vi "test compare float.vi"(8 "error in (no error)":errorcluster, 11 "VI Tester Test in":refnum<class "VI Tester Test 14.lvclass">) -> (0 "error out":errorcluster, 3 "VI Tester Test out":refnum<class "VI Tester Test 14.lvclass">)   [LabVIEW 2020, in "VI Tester Test 14.lvclass"]
uses:
  VI Tester Test 14.lvclass
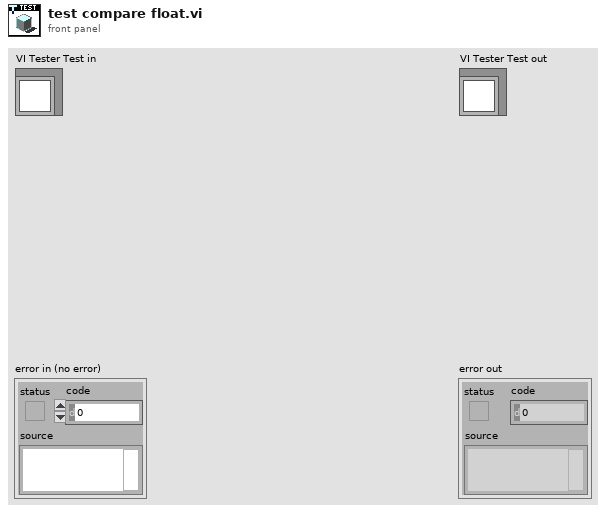
[diagram p1: front panel]
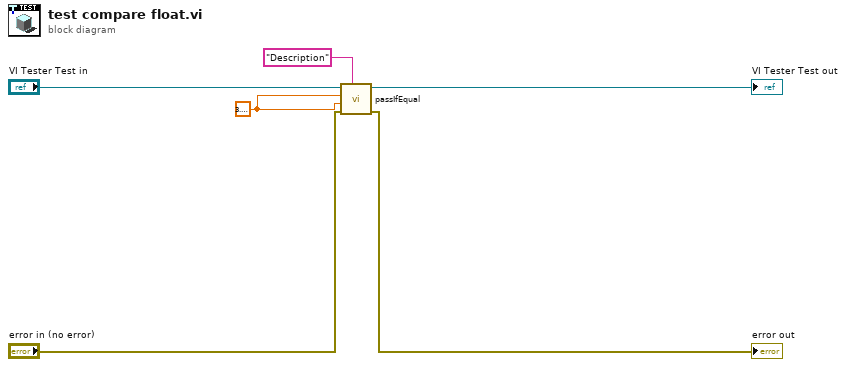
[diagram p0: block diagram]
diagram:
  w4 = 3.141592653589793
  n1 = call-dynamic "passIfEqual.vi"("custom report message (\"\")"="Description" ("custom report message (\"\")"), "error in (no error)"="error in (no error)", "y"=w4, "x"=w4, "TestCase in"="VI Tester Test in") -> ("error out"=→"error out":errorcluster, "TestCase out"=→"VI Tester Test out":refnum<class "VI Tester Test 14.lvclass">)  [unwired: 5 in]
